vi "Throw Path Parsing Error.vi"(8 "error in":errorcluster) -> (0 "error out":errorcluster)   [LabVIEW 2017, in "Variant Data Manipulation.lvlib"]
uses:
  Variant Data Manipulation.lvlib
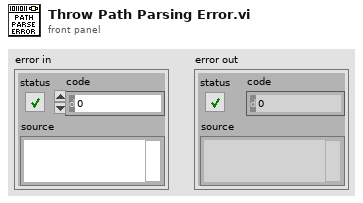
[diagram p1: front panel]
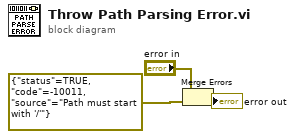
[diagram p0: block diagram]
diagram:
  n1 = Merge Errors("error in", errorcluster {"status"=TRUE, "code"=-10011, "source"="Path must start with '/'"} ("error out 2")) -> (→"error out":errorcluster)
